vi "CurlingRobot_DrivingController_DGIST_ver.Manual.vi"() -> ()   [LabVIEW 2015]
uses:
  <vilib>/myRIO/Express VI/Onboard IO/AO/AO Express VI.xnode
  <vilib>/myRIO/Instrument Drivers/Onboard IO/AO/typedefs/AO Reference.ctl
  <vilib>/myRIO/Instrument Drivers/Onboard IO/AO/AO.lvlib
  <vilib>/myRIO/Common/Instrument Driver Framework/Utilities/typedefs/Analog Scaling Constants List.ctl
  <vilib>/myRIO/Common/Instrument Driver Framework/Utilities/typedefs/Analog Scaling Constants.ctl
  <vilib>/myRIO/Common/Instrument Driver Framework/myRIO v1.0/AO/typedefs/AO Channels List.ctl
  <vilib>/myRIO/Common/Instrument Driver Framework/myRIO v1.0/AO/typedefs/AO Channels Enum.ctl
  <vilib>/myRIO/Common/Instrument Driver Framework/Utilities/typedefs/myRIO Generic Hardware Reference.ctl
  <vilib>/myRIO/Common/Instrument Driver Framework/Utilities/typedefs/myRIO v1.0 Reference.ctl
  <vilib>/myRIO/Common/Instrument Driver Framework/Utilities/typedefs/Generic FPGA Reference.ctl
  <vilib>/myRIO/Common/Instrument Driver Framework/Utilities/typedefs/Hardware Version Enum.ctl
  <vilib>/myRIO/Instrument Drivers/Onboard IO/AO/vis/myRIO AO Open.xnode
  <vilib>/userdefined/High Color/nirio_resource_hc.ctl
  <vilib>/myRIO/Common/Instrument Driver Framework/myRIO v1.0/AO/vis/myRIO v1.1 Open AO.vi
  <vilib>/myRIO/Common/Instrument Driver Framework/Utilities/vis/Is FPGA Ref Available.vi
  <vilib>/platform/TimedLoop/XDataNode/XDataNode.xnode
  <vilib>/Platform/TimedLoop/XDataNode/timing_clust.ctl
  <vilib>/Platform/TimedLoop/XDataNode/XDNodeRunTimeDep.lvlib
  <vilib>/Platform/TimedLoop/XDataNode/wakeup.ctl
  <vilib>/Platform/TimedLoop/XDataNode/nitl_modes.ctl
  <vilib>/myRIO/Express VI/Onboard IO/Encoder/Encoder Express VI.xnode
  <vilib>/myRIO/Common/Instrument Driver Framework/myRIO v1.0/Encoder/typedefs/Encoder Count Direction Enum.ctl
  <vilib>/myRIO/Instrument Drivers/Onboard IO/Encoder/typedefs/Encoder Reference.ctl
  <vilib>/myRIO/Instrument Drivers/Onboard IO/Encoder/Encoder.lvlib
  <vilib>/myRIO/Common/Instrument Driver Framework/myRIO v1.0/Encoder/typedefs/Encoder Channels Enum.ctl
  <vilib>/myRIO/Common/Instrument Driver Framework/myRIO v1.0/Encoder/typedefs/Encoder Signal Mode.ctl
  <vilib>/myRIO/Instrument Drivers/Onboard IO/Encoder/vis/Read.vi
  <vilib>/myRIO/Instrument Drivers/Onboard IO/Encoder/vis/myRIO Encoder Open.xnode
  <vilib>/myRIO/Common/Instrument Driver Framework/myRIO v1.0/Encoder/typedefs/Encoder Configuration v1.0.ctl
  <vilib>/myRIO/Common/Instrument Driver Framework/myRIO v1.0/Encoder/vis/myRIO v1.1 Open Encoder.vi
  <vilib>/myRIO/Common/Instrument Driver Framework/myRIO v1.0/Encoder/vis/myRIO v1.0 Configure Encoder.vi
  <vilib>/myRIO/Express VI/Onboard IO/DO/DO Express VI.xnode
  <vilib>/myRIO/Instrument Drivers/Onboard IO/DIO/typedefs/DIO Reference.ctl
  <vilib>/myRIO/Instrument Drivers/Onboard IO/DIO/DIO.lvlib
  <vilib>/myRIO/Common/Instrument Driver Framework/myRIO v1.0/DIO/typedefs/DIO Channels List.ctl
  <vilib>/myRIO/Common/Instrument Driver Framework/myRIO v1.0/DIO/typedefs/DIO Channels Enum.ctl
  <vilib>/myRIO/Instrument Drivers/Onboard IO/DIO/vis/myRIO DIO Open.xnode
  <vilib>/myRIO/Common/Instrument Driver Framework/myRIO v1.0/DIO/vis/myRIO v1.1 Open DIO.vi
  <vilib>/myRIO/Instrument Drivers/Onboard IO/I2C/I2C.lvlib
  <vilib>/myRIO/Instrument Drivers/Onboard IO/I2C/typedefs/I2C User Configuration.ctl
  <vilib>/myRIO/Instrument Drivers/Onboard IO/I2C/typedefs/I2C Transfer Rate.ctl
  <vilib>/myRIO/Instrument Drivers/Utilities/Utilities.lvlib
  <vilib>/Instr/_visa.llb/VISA Configure Serial Port (Instr).vi
  <vilib>/myRIO/Express VI/Onboard Devices/LED/LED Express VI.xnode
panel:
  in  "ratelimit band 2":dbl=0.0007
  in  "ratelimit cut 2":dbl=20.0
  in  "yaw_ratelimit 2":dbl=0.03
  out "Kt 3":dbl=0.062 format="%#_13g"
  out "Kt 2":dbl=0.062 format="%#_13g"
  in  "Yaw Cont on/off":bool
  in  "Kt":dbl=0.062 format="%#_13g"
  in  "acc m/s^2 Target":dbl=1.0
  in  "YMO 2":bool
  in  "Reset":bool
  in  "Start":bool
  in  "enable":bool
  in  "vel_target":dbl=4.0
  in  "Angle":dbl
  out "now ang":dbl
  out "resetloop2":i32
  out "reset loop":i32=141402027
  in  "system off":bool
  out "mainloop":bool
  out "reset":bool
  out "outer loop time":i32
  in  "MFC":bool
  out "Wheel R_L velocity":cluster{dbl, dbl}(graph)={-1.1e-322, -1.6252354122998597e-232}
  in  "PD_cut_rot 2":dbl=500.0
  in  "Kp_rot 3":dbl=0.01
  in  "Kd_rot 4":dbl=0.0005
  out "ang_bias remover":dbl=180.0
  out "Abs angle or gyro":dbl=-0.00531
  in  "abs gy stop Button":bool
  in  "system off":bool
  in  "reset loop":bool
  out "vel_ref_velFB_YMOO":cluster{"V_in":dbl, dbl, "DOB FB":dbl}(graph)={"V_in"=8.658658111174331e-05, -1.5e-323, "DOB FB"=-0.0}
  in  "Mass":dbl=73.0
  out "now interation":i32
  in  "ratelimit band":dbl=0.0007
  in  "ratelimit cut":dbl=20.0
  in  "yaw_ratelimit":dbl=0.03
  out "time_now":u32=1627815
  out "tq in":dbl=0.000865321600614421
  out "Tq rot in":dbl
  out "DOB FB":dbl=-0.0
  out "Tq_inMFC":T1={"Numeric Control"=0.000865321600614421, "Numeric Control"=0.000865321600614421}
  out "Tq_in":T1={"Numeric Control"=0.000865321600614421, "Numeric Control"=0.000865321600614421}
  in  "Ki_longi":dbl=0.01
  in  "Kp_longi":dbl=10.0
  out "GyrowithHPF":dbl
  in  "Wheel Radius":dbl=0.125 format="%#_13g"
  out "V_wheel":dbl=-1.5e-323
  in  "Wheel B":dbl=1.0 format="%#_13g"
  in  "Wheel J":dbl=1.0 format="%#_13g"
  out "Wheel_OmegaL":dbl=-1.6252354122998597e-232
  out "Wheel_OmegaR":dbl=-1.1e-322
  out "Sampling Time":u32(graph)=1
  in  "MFC_FB_gain":dbl=2.0
  in  "MFC_HPF_cut":dbl=1.0
  in  "gy_offset_remover cutoff":dbl=0.05
  in  "PD on":bool
  in  "Kd_rot 3":dbl=0.003
  in  "Kp_rot 2":dbl=0.5
  in  "PD_cut_rot":dbl=30.0
  in  "FF_cut":dbl=3.0
  in  "DOB on":bool
  in  "DOB_FB_cut":dbl=16.0
  in  "Bm_rot":dbl=2.1
  in  "Jm_rot":dbl=0.6
  in  "Vel_cut":dbl=30.0
  out "Z rate":i16=79
  in  "[main loop]":bool
  # "longi vel cmd"
  # "MFC"
  # "Output"
  # "Longi vel control"
  # "Longi_ratelimeter"
  # "Yaw ref"
  # "Yaw control"
  # "Yaw  rate control"
  # "Dimension values"
  # "Gyro Filter setting"
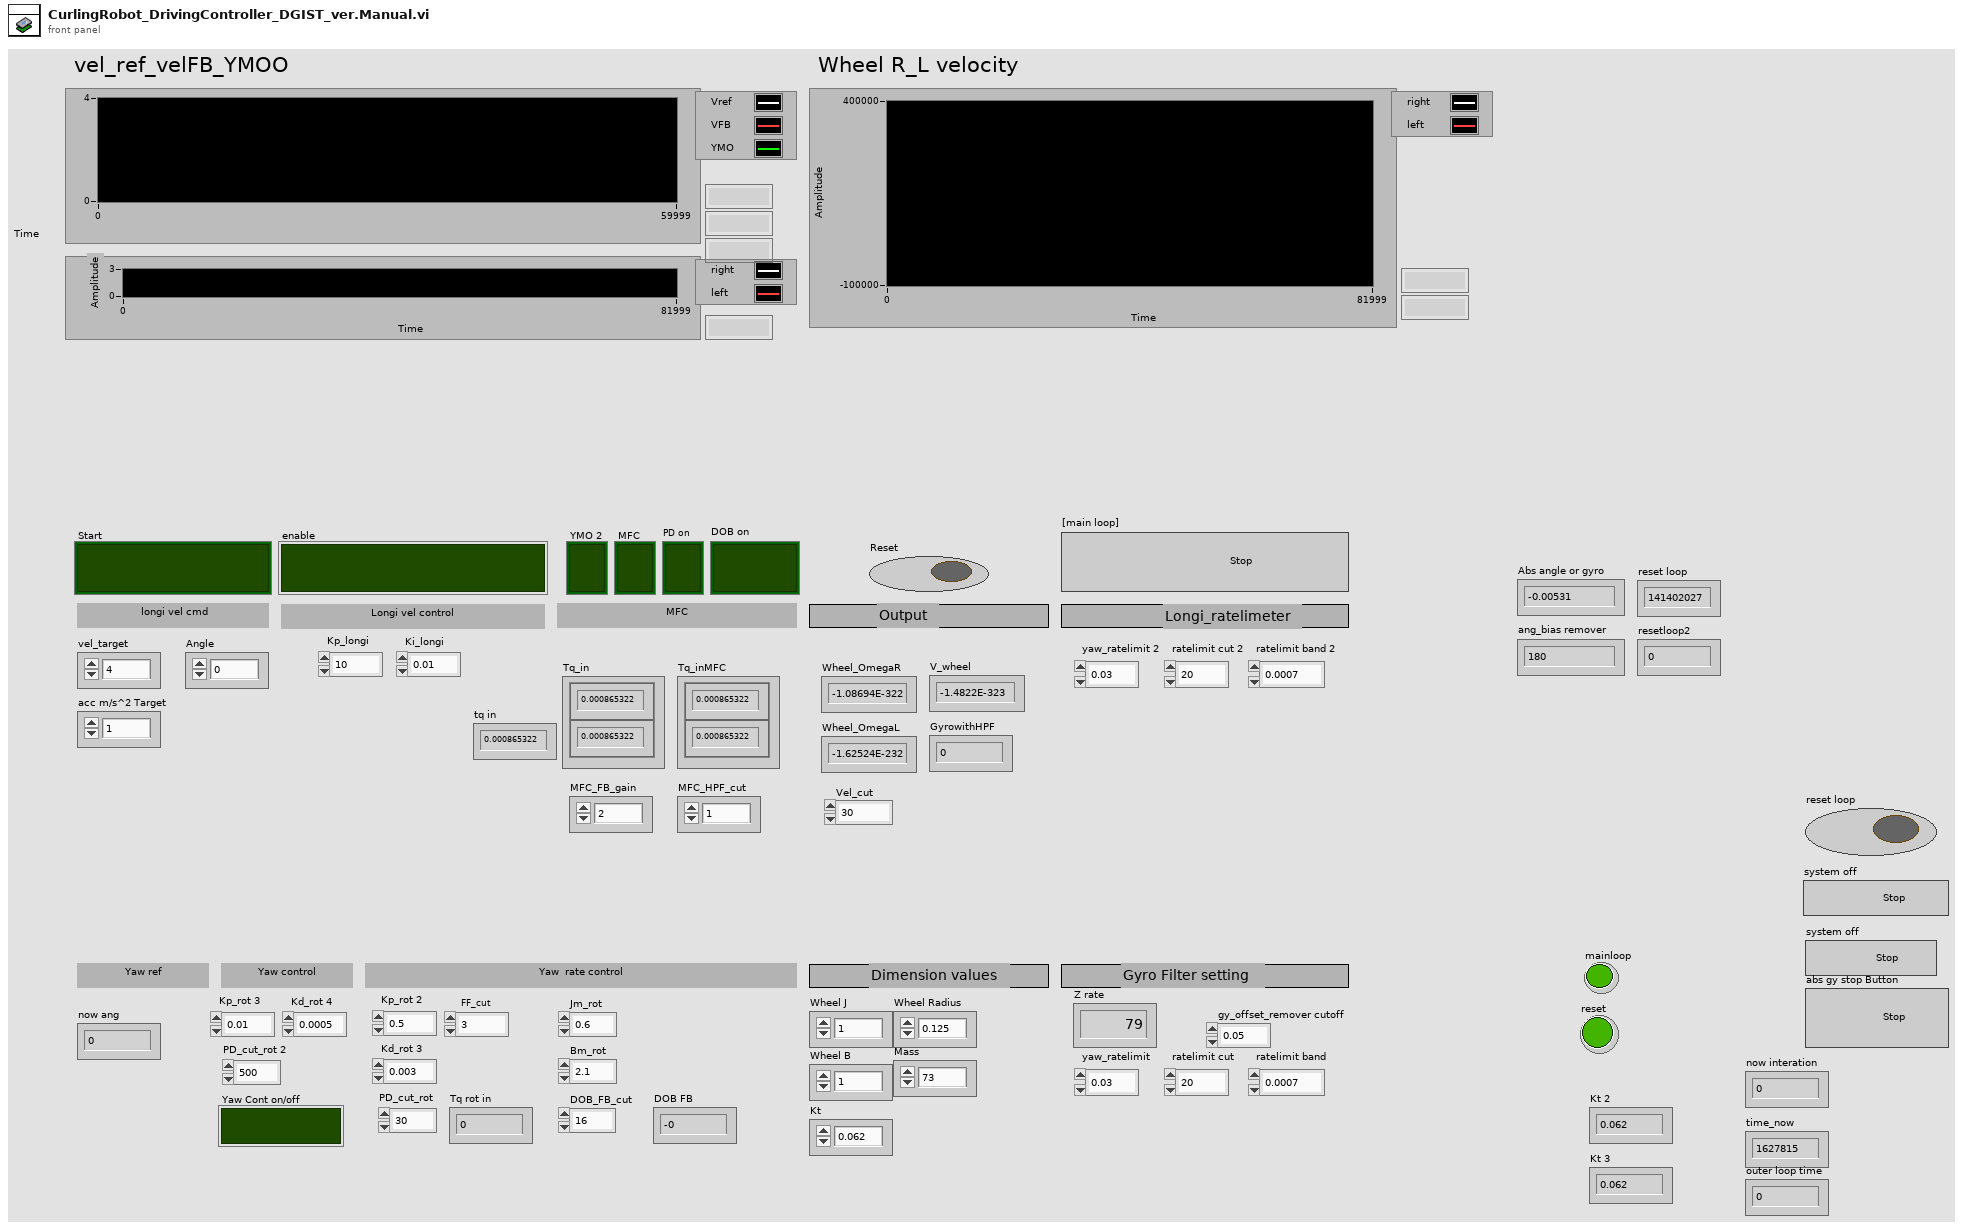
[diagram p1: front panel]
types:
  T1 = cluster{"Numeric Control":dbl, "Numeric Control":dbl}
  T2 = typedef "XDNodeRunTimeDep.lvlib/timing_clust.ctl" = cluster{"Expected End [f-1]":u64, "Actual End [f-1]":u64, "Finished Late? [f-1]":bool, "Expected End [i-1]":u64, "Actual End [i-1]":u64, "Finished Late? [i-1]":bool, "Expected Start [i]":u64, "Actual Start [i]":u64, "Expected Start [f]":u64, "Actual Start [f]":u64, "Source Name":string, "Structure Name":string, "Period":i64, "Deadline":i64, "Offset":i64, "Start":i64, "Priority":i32, "Timeout":i32, "Mode":T3, "Wakeup Reason":T4, "Error":errorcluster, "Source Type":string, "Secondary Source Type":string, "Global End Time":u64, "Global Start Time":u64, "Frame Duration":u64, "Iteration Duration":u64, "Assigned CPU":i32, "I/O Scan Engine Mode":u32}
  T3 = typedef "XDNodeRunTimeDep.lvlib/nitl_modes.ctl" = enum32{"No Change", "Process missed periods, maintain original phase", "Discard missed periods, maintain original phase", "Process missed periods, ignore original phase", "Discard missed periods, ignore original phase"}
  T4 = typedef "XDNodeRunTimeDep.lvlib/wakeup.ctl" = enum32{"Normal", "Aborted", "Asynchronous wakeup", "Timing source error", "Timed loop error", "Timeout"}
  T5 = typedef "DIO.lvlib/DIO Reference.ctl" = cluster{"myRIO Reference":T6, "DIO Channels List":T10}
  T6 = typedef "myRIO Generic Hardware Reference.ctl" = cluster{"myRIO Model":T7, "myRIO Hardware Reference":T8}
  T7 = typedef "Hardware Version Enum.ctl" = enum16{"Unknown", "myRIO-1900", "myRIO-1950", "roboRIO"}
  T8 = typedef "myRIO v1.0 Reference.ctl" = cluster{"Generic FPGA Reference":T9, "Allow multiple opens":bool}
  T9 = typedef "Generic FPGA Reference.ctl" = refnum<k20>
  T10 = typedef "DIO Channels List.ctl" = T11[]
  T11 = typedef "DIO Channels Enum.ctl" = enum16{"Not Connected", "C/DIO0", "C/DIO1", "C/DIO2", "C/DIO3", "C/DIO4", "C/DIO5", "C/DIO6", "C/DIO7", "A/DIO0", "A/DIO1", "A/DIO2", "A/DIO3", "A/DIO4", "A/DIO5", "A/DIO6", "A/DIO7", "A/DIO8", "A/DIO9", "A/DIO10", "A/DIO11", "A/DIO12", "A/DIO13", "A/DIO14", "A/DIO15", "B/DIO0", "B/DIO1", "B/DIO2", "B/DIO3", "B/DIO4", "B/DIO5", "B/DIO6", "B/DIO7", "B/DIO8", "B/DIO9", "B/DIO10", "B/DIO11", "B/DIO12", "B/DIO13", "B/DIO14", "B/DIO15", "LED0", "LED1", "LED2", "LED3", "Button0", "DIO/DIO0", "DIO/DIO1", "DIO/DIO2", "DIO/DIO3", "DIO/DIO4", "DIO/DIO5", "DIO/DIO6", "DIO/DIO7", "DIO/DIO8", "DIO/DIO9", "SPI/CS0", "SPI/CS1", "SPI/CS2", "SPI/CS3", "LED RADIO (Green)", "LED RADIO (Red)", "LED COMM (Green)", "LED COMM (Red)", "LED MODE (Green)", "LED MODE (Red)"}
  T12 = typedef "nirio_resource_hc.ctl" = tag
  T13 = typedef "Encoder.lvlib/Encoder Reference.ctl" = cluster{"myRIO Reference":T6, "Encoder Channels Enum":T14}
  T14 = typedef "Encoder Channels Enum.ctl" = enum16{"Not Connected", "C/ENC0", "C/ENC1", "A/ENC", "B/ENC", "DIO/ENC0", "DIO/ENC1", "DIO/ENC2", "DIO/ENC3", "DIO/ENC4"}
  T15 = typedef "Encoder Signal Mode.ctl" = enum16{"Quadrature phase signal", "Step and direction signal"}
  T16 = typedef "AO.lvlib/AO Reference.ctl" = cluster{"myRIO Reference":T6, "AO Channel List":T17, "AO Scaling Constant List":T19}
  T17 = typedef "AO Channels List.ctl" = T18[]
  T18 = typedef "AO Channels Enum.ctl" = enum16{"Not Connected", "AudioOut/Left", "AudioOut/Right", "C/AO0", "C/AO1", "A/AO0", "A/AO1", "B/AO0", "B/AO1"}
  T19 = typedef "Analog Scaling Constants List.ctl" = T20[]
  T20 = typedef "Analog Scaling Constants.ctl" = cluster{"LSB Weight (Volts)":dbl, "Offset (Volts)":dbl, "Signed?":bool}
  T21 = cluster{"baud rate (9600)":u32, "data bits (8)":u16, "parity (0:none)":enum16{"None", "Odd", "Even", "Mark", "Space"}, "stop bits (10: 1 bit)":u16, "flow control (0:none)":u16, "termination char\n(0xA = '\\n' = LF) ":u8, "Enable Termination\nChar (T)":bool, "timeout (10sec)":u32}
  T22 = typedef "I2C.lvlib/I2C User Configuration.ctl" = cluster{"I2C Transfer Rate":T23}
  T23 = typedef "I2C.lvlib/I2C Transfer Rate.ctl" = enum16{"Standard mode (100 kbps)", "Fast mode (400 kbps)"}
  T24 = typedef "I2C.lvlib/I2C Reference.ctl" = cluster{"myRIO Reference":T6, "I2C Channels Enum":T25, "I2C Configuration":T26}
  T25 = typedef "I2C Channels Enum.ctl" = enum16{"Not Connected", "A/I2C", "B/I2C", "I2C/I2C"}
  T26 = typedef "I2C.lvlib/I2C Configuration.ctl" = cluster{"I2C Transfer Rate":T23}
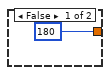
[diagram p7: hidden frame]
diagram:
  n1 = flat-sequence {
    frame #0 {
      n2 = node-c288() -> (w2:T2)  [unwired: 4 in]
      n3 = timed-loop {
        timing: w2 -> [_]
        timing-out: [_] -> w1
        i -> [w4]
        stop <- w6 stop-if-true
        w3 = 0 ("outer loop time 2")
        n4 = node-c288() -> ()  [unwired: 1 in, 1 out]
        n5 = local write "outer loop time"(w3) -> ()
        n6 = Greater?(x=w4, y=3.0) -> (0:w6:bool)
        n7 = local write "time_now"(w3) -> ()
        n8 = node-c288() -> ()  [unwired: 1 in, 1 out]
      }
      n9 = node-c288(w1) -> ()  [unwired: 1 out]
    }
    frame #1 {
      w12 = T21 {"baud rate (9600)"=38400, "data bits (8)"=8, "parity (0:none)"=enum."None", "stop bits (10: 1 bit)"=10, "flow control (0:none)"=0, "termination char\n(0xA = '\\n' = LF) "=10, "Enable Termination\nChar (T)"=TRUE, "timeout (10sec)"=10000}  # VISA Configuration
      w11 = refnum<visa-resource-name> "ASRL1::INSTR"  # VISA resource name in
      w32 = T22 {"I2C Transfer Rate"=enum."Fast mode (400 kbps)"}  # I2C bus speed
      w31 = tag "A/I2C"  # I2C channel
      w38 = u8 105  # PmodGYRO address
      # "Enable INT1 & \"data ready\" interrupt on INT2 pin"
      # "CTRL_REG3"
      # "Select HPF cutoff frequency"
      # "CTRL_REG2"
      # "Output select for LPF/HPF (both bypassed)"
      # "CTRL_REG5"
      # "Initialize device"
      # "Select data rate and enable measurements"
      # "Z-axis HI threshold"
      # "Enable interrupt on Z greater than HI threshold"
      # "CTRL_REG1"
      # "INT1_THS_ZH"
      # "INT1_CFG"
      # "Full scale setting = 100 dps"
      # "CTRL_REG4"
      # "register / data"
      n10 = while {
        i -> [w41]
        stop <- "system off" stop-if-true
        n11 = feedback #1(0) -> (w43:i32)
        n12 = case shown="False" "Reset" {
          tunnel: [w60 w61] -> w45
          tunnel: w41 -> [w60 _]
          tunnel: w43 -> [_ w61]
          frame False {
          }
          frame True {
          }
        }
        n13 = feedback-in #1(w45) -> ()
        n14 = Subtract(x=w41, y=w45) -> (x-y=w46:i32)
        "resetloop2" <- w46
        n15 = case shown="True" "Reset" {
          tunnel: w46 -> [_ w59]
          frame False {
          }
          frame True {
            n16 = Divide(x=w59, y=10000) -> (x/y=w51:dbl)
            n17 = Greater?(x=w51, y=1.0) -> (0:w54:bool)
            n18 = Greater?(x=w51, y=2.0) -> (0:w49:bool)
            n19 = Less?(x=w51, y=3.0) -> (x < y?=w53:bool)
            n20 = Less?(x=w51, y=4.0) -> (x < y?=w48:bool)
            n21 = And(x=w49, y=w48) -> (x .and. y?=w47:bool)
            "mainloop" <- w47
            n22 = local write "[main loop]"(w47) -> ()
            n23 = And(x=w54, y=w53) -> (x .and. y?=w52:bool)
            "reset" <- w52
            n24 = local write "reset loop"(w52) -> ()
            "outer loop time" <- w59
          }
        }
        "reset loop" <- w41
      }
      n25 = Unbundle By Name(w12) -> ("Enable Termination\nChar (T)"=w15:bool, "termination char\n(0xA = '\\n' = LF)"=w16:u8, "timeout (10sec)"=w17:u32, "baud rate (9600)"=w22:u32, "data bits (8)"=w21:u16, "parity (0:none)"=w20:enum16{"None", "Odd", "Even", "Mark", "Space"}, "stop bits (10: 1 bit)"=w19:u16, "flow control (0:none)"=w18:u16)
      n26 = call <vilib>:"Open.vi"("Channel Name"=w31) -> ("error out"=w34:errorcluster, "I2C Ref Out"=w33:T24)  [unwired: 9 in]
      n27 = node-c288() -> (w24:T2)  [unwired: 4 in]
      n28 = call-poly "VISA Configure Serial Port"("VISA resource name"=w11, "timeout (10sec)"=w17, "termination char\n(0xA = '\\n' = LF)"=w16, "Enable Termination\nChar (T)"=w15, "baud rate (9600)"=w22, "data bits (8)"=w21, "parity (0:none)"=w20, "stop bits (10: 1 bit)"=w19, "flow control (0:none)"=w18) -> ("VISA resource name out"=w13:refnum<visa-resource-name>, "error out"=w14:errorcluster)  [unwired: 5 in]
      n29 = call <vilib>:"Configure.vi"("error in (no error)"=w34, "I2C User Configuration"=w32, "I2C Ref In"=w33) -> ("error out"=w37:errorcluster, "I2C Ref Out"=w36:T24)  [unwired: 7 in]
      n30 = timed-loop {
        tunnel: w13 -> [w72]
        tunnel: w14 -> [w71]
        timing: w24 -> [_]
        timing-out: [_] -> w23
        stop <- "abs gy stop Button" stop-if-true
        w69 = u32 128  # 바이트 카운트
        n31 = node-c288() -> ()  [unwired: 1 in, 1 out]
        n32 = property class="Instr" props=["Serial Settings:Number of Bytes at Serial Port"](reference=w72) -> (reference out=w70:refnum<visa-resource-name>)  [unwired: 1 in, 2 out]
        n33 = call <vilib>:"Space Constant.vi"() -> ("String"=w65:string)
        n34 = VISA Read(VISA resource name=w70, byte count=w69, error in (no error)=w71) -> (read buffer=w68:string)  [unwired: 3 out]
        n35 = call <vilib>:"Trim Whitespace.vi"("string"=w68) -> ("trimmed string"=w67:string)  [unwired: 1 in]
        n36 = Match Pattern(string=w67, regular expression=w65) -> (before substring=w66:string)  [unwired: 1 in, 3 out]
        n37 = call <vilib>:"Trim Whitespace.vi"("string"=w66) -> ("trimmed string"=w64:string)  [unwired: 1 in]
        n38 = Fract/Exp String To Number(string=w64) -> (number=→"Abs angle or gyro":dbl)  [unwired: 3 in, 1 out]
        n39 = node-c288() -> ()  [unwired: 1 in, 1 out]
      }
      n40 = for {
        tunnel: [w696] -> w28
        tunnel: [w695] -> w27
        tunnel: [w691] -> w29
        tunnel: u8[][] [[34, 136], [35, 0], [48, 32], [54, 80], [36, 0], [33, 9], [32, 15]] ("Bytes to Write") -> [w694] mode=indexing
        tunnel: w36 -> [w693]
        tunnel: w37 -> [w692]
        tunnel: w38 -> [w691]
        n41 = call <vilib>:"Write.vi"("error in (no error)"=w692, "Bytes to Write"=w694, "Slave Address (7-bit)"=w691, "I2C Ref In"=w693) -> ("error out"=w696:errorcluster, "I2C Ref Out"=w695:T24)  [unwired: 6 in]
      }
      n42 = node-c288() -> (w26:T2)  [unwired: 4 in]
      n43 = node-c288(w23) -> ()  [unwired: 1 out]
      n44 = timed-loop {
        tunnel: w27 -> [w81]
        tunnel: w28 -> [w80]
        tunnel: w29 -> [w78]
        tunnel: [w79] -> w30
        timing: w26 -> [_]
        timing-out: [_] -> w25
        stop <- "system off" stop-if-true
        # "Integrate rate to obtain position"
        n45 = node-c288() -> ()  [unwired: 1 in, 1 out]
        n46 = case shown="False" "reset loop" {
          tunnel: w81 -> [w88 _]
          tunnel: w80 -> [w87 w688]
          tunnel: [w86 w688] -> w79
          tunnel: w78 -> [w85 _]
          frame False {
            n47 = node-c288() -> (w90:T2)  [unwired: 4 in]
            n48 = timed-loop {
              timing: w90 -> [_]
              timing-out: [_] -> w89
              tunnel: w88 -> [w202]
              tunnel: w87 -> [w201]
              tunnel: [w199] -> w86
              tunnel: w85 -> [w200]
              i -> [w284]
              stop <- "[main loop]" stop-if-true
              w157 = 0.0
              w192 = 0.0
              w218 = 0.0993 ("y")
              w279 = 0.0
              w408 = 0.001 ("input variable")
              w339 = 0.0 ("y0")
              w432 = 0.001 ("input variable")
              # "Longi velocity rate limiter"
              # "rated limiter"
              # "When stoppping LPF"
              # "angle limit +-90"
              # "To make zero angle"
              # "YR_ref"
              # "Read three 16-bit gyroscope values:\nWrite the address of the first register with MSB set to enable auto-indexing and then read six bytes"
              # "Format the six bytes into three 16-bit integers"
              # "calculatefixed offset"
              # "Rate limiter"
              # "rated limiter"
              # "save Drive time"
              # "when button start and stop within dive time automatly"
              # "Data saving"
              # "Longi velocity Plan"
              # "Longitudinal PI  controller"
              # "V longi FB"
              # "Tq longi in"
              # "Vel output"
              # "Tq rot in"
              # "Tq rot in"
              # "Gyro FB"
              # "Tq rot in"
              # "DOB FB"
              # "FF"
              # "Gyro FB"
              # "YMObser"
              # "Jacobian Robot to Wheel\nAnd (YMO FF FB) On off"
              # "YMO controller"
              # "Jacobian Wheel to robot"
              # "Wheel MFC controller"
              # "MFC_HPF"
              # "MFC controller ModelEuler not Tustin"
              # "Tq_Right"
              # "Tq_Left"
              # "Time derivative of enc to gel wheel vel"
              # "Wheel encoder gear ratio, encoder"
              # "MFC_HPF"
              # "MFC controller ModelEuler not Tustin"
              # "Rot PD  controller"
              # "gear ratio"
              # "gear ratio"
              n49 = node-c288() -> ()  [unwired: 1 in, 1 out]
              n50 = local read "ang_bias remover"() -> (w176:dbl)
              n51 = local read "now interation"() -> (w163:i32)
              n52 = local read "now interation"() -> (w234:i32)
              n53 = Greater?(x=w163, y=15000) -> (0:w153:bool)
              n54 = Greater?(x=w163, y=14000) -> (0:w149:bool)
              n55 = Greater?(x=w163, y=16000) -> (0:w154:bool)
              n56 = formula code="float phi_cmd;\nif (ref_phi >= 70)\nphi_cmd = 70;\nelse if (ref_phi <= -70)\nphi_cmd = -70;\nelse\nphi_cmd = ref_phi;"("ref_phi"="Angle") -> ("phi_cmd"=w179:dbl)
              n57 = Divide(x=w234, y=u32 1000) -> (x/y=w135:dbl)
              n58 = feedback #2(w157) -> (w160:dbl)
              n59 = case shown="False" w149 {
                tunnel: w176 -> [w487 _]
                tunnel: [w487 w488] -> w150
                tunnel: w160 -> [_ w488]
                frame False {
                }
                frame True {
                }
              }
              n60 = feedback-in #2(w150) -> ()
              n61 = feedback #3(w157) -> (w158:dbl)
              n62 = case shown="False" w154 {
                tunnel: w176 -> [w483 _]
                tunnel: [w483 w484] -> w156
                tunnel: w158 -> [_ w484]
                frame False {
                }
                frame True {
                }
              }
              n63 = feedback-in #3(w156) -> ()
              n64 = feedback #4(w157) -> (w159:dbl)
              n65 = case shown="False" w153 {
                tunnel: w176 -> [w485 _]
                tunnel: [w485 w486] -> w155
                tunnel: w159 -> [_ w486]
                frame False {
                }
                frame True {
                }
              }
              n66 = feedback-in #4(w155) -> ()
              n67 = Compound Arithmetic op=ADD(w158, w159, w160) -> (w161:dbl)
              n68 = Divide(x=w161, y=3.0) -> (x/y=w164:dbl)
              n69 = Subtract(x=w176, y=w164) -> (x-y=w178:dbl)
              "now ang" <- w178
              n70 = formula code="float phi;\nif (sensor > 90 && sensor <=270)\nphi = 180-sensor;\nelse if (sensor >270)\nphi = sensor - 360;\nelse\nphi = sensor;"("sensor"=w178) -> ("phi"=w177:dbl)
              n71 = Negate(x=w177) -> (-x=w182:dbl)
              n72 = Bundle(w179, w182) -> ()  [unwired: 1 in, 1 out]
              n73 = Subtract(x=w179, y=w182) -> (x-y=w180:dbl)
              n74 = Add(x=w180, y=0.0) -> (x+y=w181:dbl)
              n75 = feedback #5(0.0) -> (w169:dbl)
              n76 = feedback-in #5(w181) -> ()
              n77 = call <vilib>:"Write Read.vi"("Byte Count"=u32 6, "error in (no error)"=w201, "Bytes to Write"=u8[] [168], "Slave Address (7-bit)"=w200, "I2C Ref In"=w202) -> ("error out"=w199:errorcluster, "Bytes Read"=w217:u8[])  [unwired: 3 in, 1 out]
              n78 = Index Array "Index Array"(array=w217) -> (element #1=w212:u8, element #2=w211:u8, element #3=w210:u8, element #4=w209:u8, element #5=w208:u8, element #6=w207:u8)  [unwired: 6 in]
              n79 = Multiply(x="PD_cut_rot 2", y=6.283185307179586) -> (x*y=w166:dbl)
              n80 = Join Numbers(hi=w211, lo=w212) -> ((hi.lo)=w215:u16)
              n81 = Join Numbers(hi=w209, lo=w210) -> ((hi.lo)=w214:u16)
              n82 = Join Numbers(hi=w207, lo=w208) -> ((hi.lo)=w213:u16)
              n83 = Reciprocal(x=w166) -> (1/x=w167:dbl)
              n84 = feedback #6(0.0) -> (w173:dbl)
              n85 = formula code="float F,A,B,C,ykd,ykp,y0;\nF=2*tau+T;\nA=(2*Kd_rot)/F;\nB=(-2*Kd_rot)/F;\nC=(2*tau-T)/F;\nykd=A*u0+B*u1+C*y1;\nykp=Kp_rot*u0;\ny0=ykp+ykd;"("tau"=w167, "u0"=w181, "u1"=w169, "y1"=w173, "T"=0.001 ("input variable"), "Kp_rot"="Kp_rot 3", "Kd_rot"="Kd_rot 4") -> ("y0"=w183:dbl)
              n86 = feedback-in #6(w183) -> ()
              n87 = To Word Integer(number=w215) -> ()  [unwired: 1 out]
              n88 = To Word Integer(number=w214) -> ()  [unwired: 1 out]
              n89 = To Word Integer(number=w213) -> (16bit integer=w216:i16)
              "Z rate" <- w216
              n90 = Add(x=0.0, y=w183) -> (x+y=w123:dbl)
              n91 = feedback #7(0.0) -> (w272:dbl)
              n92 = case shown="True" "Start" {
                tunnel: w135 -> [w540 _]
                tunnel: [w540 w541] -> w271
                tunnel: w272 -> [_ w541]
                frame False {
                }
                frame True {
                }
              }
              n93 = feedback-in #7(w271) -> ()
              n94 = Divide(x=w216, y=65535.0 ("gyroscale")) -> (x/y=w203:dbl)
              n95 = Subtract(x=w135, y=w271) -> (x-y=w131:dbl)
              n96 = formula code="float V_now;\nV_now=acc_d*t;\n\nif (V_now < V_targ && V_targ >= 0)\nV_in=V_now;\nelse if (V_targ < 0 && -V_now > V_targ )\nV_in=-V_now;\nelse \nV_in=V_targ;"("V_targ"="vel_target", "acc_d"="acc m/s^2 Target", "t"=w131) -> ("V_in"=w239:dbl)
              n97 = Select(t=w123, s="Yaw Cont on/off", f=0.0) -> (s? t:f=w122:dbl)
              n98 = feedback #8(0.0 ("V_in")) -> (w246:dbl)
              n99 = feedback-in #8(w239) -> ()
              n100 = Multiply(x=0.1, y=6.283185307179586) -> (x*y=w243:dbl)
              n101 = Reciprocal(x=w243) -> (1/x=w247:dbl)
              n102 = Multiply(x="PD_cut_rot", y=6.283185307179586) -> (x*y=w383:dbl)
              n103 = feedback #9(0.0) -> (w244:dbl)
              n104 = formula code="float F,A,B,C,y0;\nF=2*tau+T;\nA=(2*a+b*T)/F;\nB=(b*T-2*a)/F;\nC=(2*tau-T)/F;\ny0=A*u0+B*u1+C*y1;"("tau"=w247, "u0"=w239, "u1"=w246, "y1"=w244, "T"=0.001 ("input variable"), "a"=0.0 ("input variable"), "b"=1.0 ("input variable")) -> ("y0"=w236:dbl)
              n105 = case shown="False" "Start" {
                tunnel: [w538 w539] -> w118
                tunnel: w239 -> [_ w539]
                tunnel: w236 -> [w538 _]
                frame False {
                }
                frame True {
                }
              }
              n106 = feedback-in #9(w236) -> ()
              n107 = feedback #10(0.0) -> (w380:dbl)
              n108 = local read "DOB FB"() -> (w119:dbl)
              n109 = Reciprocal(x=w383) -> (1/x=w382:dbl)
              n110 = Multiply(x="FF_cut", y=6.283185307179586) -> (x*y=w405:dbl)
              n111 = feedback #11(0.0 ("gy_z[]")) -> (w393:dbl)
              n112 = feedback-in #11(w122) -> ()
              n113 = Reciprocal(x=w405) -> (1/x=w403:dbl)
              n114 = local read "Jm_rot"() -> (w314:dbl)
              n115 = feedback #12(0.0) -> (w108:dbl)
              n116 = Divide(x=w314, y=w218) -> (x/y=w313:dbl)
              n117 = local read "Bm_rot"() -> (w312:dbl)
              n118 = feedback #13(0.0) -> (w306:dbl)
              n119 = Divide(x=w312, y=w218) -> (x/y=w311:dbl)
              n120 = Multiply(x="ratelimit cut 2", y=6.283185307179586) -> (x*y=w106:dbl)
              n121 = Reciprocal(x=w106) -> (1/x=w105:dbl)
              n122 = feedback #14(0.0 ("gy_z[]")) -> (w402:dbl)
              n123 = formula code="float F,A,B,C,y0;\nF=2*tau+T;\nA=(2*a+b*T)/F;\nB=(b*T-2*a)/F;\nC=(2*tau-T)/F;\ny0=A*u0+B*u1+C*y1;"("tau"=w403, "u0"=w122, "u1"=w393, "y1"=w402, "T"=0.001 ("input variable"), "a"=w313, "b"=w311) -> ("y0"=w374:dbl)
              n124 = feedback-in #14(w374) -> ()
              n125 = feedback #15() -> (w375:dbl)  [unwired: 1 in]
              n126 = feedback #16(0.0) -> (w103:dbl)
              n127 = feedback #17(0.0 ("gy_ratelimit")) -> (w110:dbl)
              n128 = xnode "Digital output (1 sample)"("C/DIO1 (DIO1)"="enable") -> ()  [unwired: 1 in, 1 out]
              n129 = xnode "Left encoder"() -> ("Counter Value"=w139:i32)  [unwired: 2 in, 3 out]
              n130 = xnode "Encoder"() -> ("Counter Value"=w145:i32)  [unwired: 2 in, 3 out]
              n131 = Negate(x=w139) -> (-x=w138:i32)
              n132 = Negate(x=w145) -> (-x=w144:i32)
              n133 = Multiply(x=w138, y=6.283185307179586) -> (x*y=w443:dbl)
              n134 = Negate(x=w144) -> (-x=w441:i32)
              n135 = Divide(x=w443, y=32768.0) -> (x/y=w425:dbl)
              n136 = Multiply(x=w441, y=6.283185307179586) -> (x*y=w446:dbl)
              n137 = feedback #18(0.0 ("f")) -> (w224:dbl)
              n138 = Multiply(x=2.0 ("y"), y=w224) -> (x*y=w226:dbl)
              n139 = Divide(x=w446, y=32768.0) -> (x/y=w342:dbl)
              n140 = feedback #19(0.0) -> (w410:dbl)
              n141 = feedback #20(0.0 ("gy_z[]")) -> (w407:dbl)
              n142 = local read "Wheel Radius"() -> (w297:dbl)
              n143 = Bundle(w342, w425) -> (w422:cluster{dbl, dbl})  [unwired: 1 in]
              n144 = feedback #21(0.0 ("f")) -> (w222:dbl)
              n145 = Multiply(x=2.0 ("y"), y=w222) -> (x*y=w221:dbl)
              n146 = local read "Kt"() -> (w125:dbl)
              "Kt 3" <- w125
              n147 = feedback #22(0.0 ("gy_ratelimit")) -> (w266:dbl)
              n148 = local read "now interation"() -> (w134:i32)
              n149 = Divide(x=w422, y=8.0) -> (x/y=w296:cluster{dbl, dbl})
              n150 = Multiply(x=w296, y=w297) -> (x*y=w116:cluster{dbl, dbl})
              n151 = Divide(x="Jm_rot", y=w125) -> (x/y=w401:dbl)
              n152 = Multiply(x="DOB_FB_cut", y=6.283185307179586) -> (x*y=w411:dbl)
              n153 = Unbundle(w116) -> ()  [unwired: 2 out]
              n154 = Reciprocal(x=w411) -> (1/x=w413:dbl)
              n155 = feedback #23(0.0) -> (w259:dbl)
              n156 = feedback #24(0.0) -> (w436:dbl)
              n157 = feedback-in #24(w342) -> ()
              n158 = Divide(x="Bm_rot", y=w125) -> (x/y=w400:dbl)
              n159 = feedback #25(0.0) -> (w429:dbl)
              n160 = feedback-in #25(w425) -> ()
              n161 = feedback #26(0.0) -> (w328:dbl)
              n162 = feedback #27(0.0) -> (w353:dbl)
              n163 = local read "Abs angle or gyro"() -> (w187:dbl)
              n164 = Multiply(x="MFC_HPF_cut", y=6.283185307179586) -> (x*y=w355:dbl)
              n165 = Multiply(x="ratelimit cut", y=6.283185307179586) -> (x*y=w262:dbl)
              n166 = Reciprocal(x=w355) -> (1/x=w322:dbl)
              n167 = Greater?(x=w134, y=2000) -> (0:w197:bool)
              n168 = Greater?(x=w134, y=12000) -> (0:w195:bool)
              n169 = Reciprocal(x=w262) -> (1/x=w261:dbl)
              n170 = Multiply(x="Vel_cut", y=6.283185307179586) -> (x*y=w434:dbl)
              n171 = feedback #28(0.0) -> (w409:dbl)
              n172 = feedback #29(0.0) -> (w406:dbl)
              n173 = Multiply(x="Vel_cut", y=6.283185307179586) -> (x*y=w439:dbl)
              n174 = Reciprocal(x=w434) -> (1/x=w431:dbl)
              n175 = Reciprocal(x=w439) -> (1/x=w438:dbl)
              n176 = feedback #30(0.0) -> (w264:dbl)
              n177 = feedback #31(0.0) -> (w361:dbl)
              n178 = feedback-in #31(w203) -> ()
              n179 = feedback #32(0.0) -> (w391:dbl)
              n180 = feedback #33(w192) -> (w194:dbl)
              n181 = case shown="True" w197 {
                tunnel: w187 -> [w501 _]
                tunnel: [w501 w502] -> w188
                tunnel: w194 -> [_ w502]
                frame False {
                }
                frame True {
                }
              }
              n182 = feedback-in #33(w188) -> ()
              n183 = Boolean To (0,1)(Boolean="DOB on") -> (0, 1=w397:i16)
              n184 = Multiply(x=w397, y=w391) -> (x*y=w307:dbl)
              "DOB FB" <- w307
              n185 = feedback #34(w339) -> (w430:dbl)
              n186 = formula code="y0=(2*(u0-u1)-(T-2*Tau)*y1)/(T+2*Tau);"("Tau"=w431, "u0"=w425, "u1"=w429, "y1"=w430, "T"=w432) -> ("y0"=w426:dbl)
              n187 = feedback-in #34(w426) -> ()
              n188 = feedback #35(w192) -> (w193:dbl)
              n189 = case shown="False" w195 {
                tunnel: w187 -> [w499 _]
                tunnel: [w499 w500] -> w189
                tunnel: w193 -> [_ w500]
                frame False {
                }
                frame True {
                }
              }
              n190 = feedback-in #35(w189) -> ()
              n191 = feedback #36(w339) -> (w437:dbl)
              n192 = formula code="y0=(2*(u0-u1)-(T-2*Tau)*y1)/(T+2*Tau);"("Tau"=w438, "u0"=w342, "u1"=w436, "y1"=w437, "T"=w432) -> ("y0"=w341:dbl)
              n193 = feedback-in #36(w341) -> ()
              n194 = feedback #37(0.0 ("y0")) -> (w330:dbl)
              n195 = feedback #38(0.0 ("y0")) -> (w351:dbl)
              n196 = Tick Count (ms)() -> (millisecond timer value=w344:u32)
              "time_now" <- w344
              n197 = Multiply(x="gy_offset_remover cutoff", y=6.283185307179586) -> (x*y=w366:dbl)
              n198 = feedback #39() -> (w343:u32)  [unwired: 1 in]
              n199 = feedback-in #39(w344) -> ()
              n200 = Subtract(x=w344, y=w343) -> (x-y=w115:u32)
              "Sampling Time" <- w115
              n201 = Reciprocal(x=w366) -> (1/x=w288:dbl)
              n202 = feedback #40(0.0) -> (w359:dbl)
              n203 = local read "Kt"() -> (w124:dbl)
              "Kt 2" <- w124
              n204 = feedback #41(0.0) -> (w334:dbl)
              n205 = Greater?(x=w134, y=13000) -> (0:w190:bool)
              n206 = Bundle("y0"=w341, "y0"=w426) -> (w340:cluster{"y0":dbl, "y0":dbl})  [unwired: 1 in]
              n207 = Divide(x=w340, y=8.0) -> (x/y=w112:cluster{"y0":dbl, "y0":dbl})
              "Wheel R_L velocity" <- w112
              n208 = case shown="True" w190 {
                tunnel: w189 -> [_ w498]
                tunnel: [180 w494] -> w186
                tunnel: w188 -> [_ w497]
                tunnel: w187 -> [_ w490]
                tunnel: w134 -> [_ w492]
                frame False {
                }
                frame True {
                  n209 = Subtract(x=w498, y=w497) -> (x-y=w496:dbl)
                  n210 = Divide(x=w496, y=10000) -> (x/y=w493:dbl)
                  n211 = Multiply(x=w493, y=w492) -> (x*y=w491:dbl)
                  n212 = Subtract(x=w490, y=w491) -> (x-y=w494:dbl)
                }
              }
              "ang_bias remover" <- w186
              n213 = feedback #42(0.0) -> (w365:dbl)
              n214 = formula code="float F,A,B,C,y0;\nF=2*tau+T;\nA=(2*a+b*T)/F;\nB=(b*T-2*a)/F;\nC=(2*tau-T)/F;\ny0=A*u0+B*u1+C*y1;"("tau"=w288, "u0"=w203, "u1"=w361, "y1"=w365, "T"=0.001 ("input variable"), "a"=0.0 ("input variable"), "b"=1.0 ("input variable")) -> ("y0"=w267:dbl)
              n215 = feedback-in #42(w267) -> ()
              n216 = Less?(x=w115, y=1.1) -> (x < y?=w113:bool)
              n217 = Unbundle(w112) -> ("y0"=→"Wheel_OmegaR":dbl, "y0"=→"Wheel_OmegaL":dbl)
              n218 = Unbundle(w296) -> ()  [unwired: 2 out]
              n219 = xnode "LED"("LED3"=w113) -> ()  [unwired: 1 in, 1 out]
              n220 = Greater?(x=w284, y=21000) -> (0:w283:bool)
              n221 = Greater?(x=w284, y=20000) -> (0:w289:bool)
              n222 = Greater?(x=w284, y=22000) -> (0:w282:bool)
              n223 = feedback #43(0.0 ("y0")) -> (w360:dbl)
              n224 = feedback #44(0.0 ("y0")) -> (w333:dbl)
              n225 = local read "Wheel_OmegaR"() -> (w111:dbl)
              n226 = local read "Wheel_OmegaL"() -> (w91:dbl)
              n227 = feedback #45(w279) -> (w276:dbl)
              n228 = case shown="False" w289 {
                tunnel: w267 -> [w546 _]
                tunnel: [w546 w547] -> w287
                tunnel: w276 -> [_ w547]
                frame False {
                }
                frame True {
                }
              }
              n229 = feedback-in #45(w287) -> ()
              n230 = feedback #46(w279) -> (w278:dbl)
              n231 = case shown="False" w282 {
                tunnel: w267 -> [w542 _]
                tunnel: [w542 w543] -> w280
                tunnel: w278 -> [_ w543]
                frame False {
                }
                frame True {
                }
              }
              n232 = feedback-in #46(w280) -> ()
              n233 = feedback #47(w279) -> (w277:dbl)
              n234 = case shown="False" w283 {
                tunnel: w267 -> [w544 _]
                tunnel: [w544 w545] -> w281
                tunnel: w277 -> [_ w545]
                frame False {
                }
                frame True {
                }
              }
              n235 = feedback-in #47(w281) -> ()
              n236 = Compound Arithmetic op=ADD(w278, w277, w276) -> (w275:dbl)
              n237 = Add(x=w111, y=w91) -> (x+y=w318:dbl)
              n238 = Divide(x=w275, y=3.0) -> (x/y=w250:dbl)
              n239 = Subtract(x=w203, y=w250) -> (x-y=w233:dbl)
              n240 = formula code="float rate;\nrate=gy-gy_r1;\nif (rate > limit)\ngy_ratelimit=gy_r1+limit;\nelse if (rate < -limit)\ngy_ratelimit=gy_r1+(-limit);\nelse\ngy_ratelimit=gy;"("gy"=w233, "gy_r1"=w266, "limit"="yaw_ratelimit") -> ("gy_ratelimit"=w249:dbl)
              n241 = feedback-in #22(w249) -> ()
              n242 = feedback-in #23(w249) -> ()
              n243 = formula code="float F,A,B,C,y0;\nF=2*tau+T;\nA=(2*a+b*T)/F;\nB=(b*T-2*a)/F;\nC=(2*tau-T)/F;\ny0=A*u0+B*u1+C*y1;"("tau"=w261, "u0"=w249, "u1"=w259, "y1"=w264, "T"=0.001 ("input variable"), "a"=0.0 ("input variable"), "b"=1.0 ("input variable")) -> ("y0"=w254:dbl)
              n244 = feedback-in #30(w254) -> ()
              n245 = formula code="float band_ratelim;\n\nif (gy_ratelim < gy_band && gy_ratelim > -gy_band)\nband_ratelim=0;\nelse\nband_ratelim=gy_ratelim;"("gy_ratelim"=w254, "gy_band"="ratelimit band") -> ("band_ratelim"=w137:dbl)
              "GyrowithHPF" <- w137
              n246 = Subtract(x=w122, y=w137) -> (x-y=w379:dbl)
              n247 = feedback-in #10(w379) -> ()
              n248 = formula code="float F,A,B,C,ykd,ykp,y0;\nF=2*tau+T;\nA=(2*Kd_rot)/F;\nB=(-2*Kd_rot)/F;\nC=(2*tau-T)/F;\nykd=A*u0+B*u1+C*y1;\nykp=Kp_rot*u0;\ny0=ykp+ykd;"("tau"=w382, "u0"=w379, "u1"=w380, "y1"=w375, "T"=0.001 ("input variable"), "Kp_rot"="Kp_rot 2", "Kd_rot"="Kd_rot 3") -> ("y0"=w371:dbl)
              n249 = feedback-in #15(w371) -> ()
              n250 = Select(t=w371, s="PD on", f=0.0) -> (s? t:f=w310:dbl)
              n251 = Add(x=w374, y=w310) -> (x+y=w147:dbl)
              n252 = Add(x=0.0, y=w147) -> (x+y=w146:dbl)
              n253 = Subtract(x=w146, y=w307) -> (x-y=w308:dbl)
              "Tq rot in" <- w308
              n254 = formula code="v_L=-error_YR/2;\n\nif (v_L < 16.5 && v_L > -16.5)\nv_L=v_L;\nelse if (v_L >=16.5)\nv_L=16.5;\nelse\nv_L=-16.5;\nv_R=error_YR/2;\n\nif (v_R < 16.5 && v_R > -16.5)\nv_R=v_R;\nelse if (v_R >=16.5)\nv_R=16.5;\nelse\nv_R=-16.5;"("error_YR"=w308) -> ("v_L"=w315:dbl, "v_R"=w316:dbl)
              n255 = feedback-in #19(w308) -> ()
              n256 = feedback-in #20(w137) -> ()
              n257 = formula code="float F,A,B,C,y0;\nF=2*tau+T;\nA=(2*a+b*T)/F;\nB=(b*T-2*a)/F;\nC=(2*tau-T)/F;\ny0=A*u0+B*u1+C*y1;"("tau"=w413, "u0"=w137, "u1"=w407, "y1"=w406, "T"=w408, "a"=w401, "b"=w400) -> ("y0"=w395:dbl)
              n258 = formula code="float F,A,B,C,y0;\nF=2*tau+T;\nA=(2*a+b*T)/F;\nB=(b*T-2*a)/F;\nC=(2*tau-T)/F;\ny0=A*u0+B*u1+C*y1;"("tau"=w413, "u0"=w308, "u1"=w410, "y1"=w409, "T"=w408, "a"=0.0 ("input variable"), "b"=1.0 ("input variable")) -> ("y0"=w399:dbl)
              n259 = feedback-in #28(w399) -> ()
              n260 = feedback-in #29(w395) -> ()
              n261 = Subtract(x=w395, y=w399) -> (x-y=w398:dbl)
              n262 = feedback-in #32(w398) -> ()
              n263 = Divide(x=w318, y=2.0) -> ()  [unwired: 1 out]
              n264 = Multiply(x=w91, y="Wheel Radius") -> (x*y=w93:dbl)
              "V_wheel" <- w93
              n265 = formula code="float rate;\nrate=gy-gy_r1;\nif (rate > limit)\ngy_ratelimit=gy_r1+limit;\nelse if (rate < -limit)\ngy_ratelimit=gy_r1+(-limit);\nelse\ngy_ratelimit=gy;"("gy"=w93, "gy_r1"=w110, "limit"="yaw_ratelimit 2") -> ("gy_ratelimit"=w94:dbl)
              n266 = formula code="float F,A,B,C,y0;\nF=2*tau+T;\nA=(2*a+b*T)/F;\nB=(b*T-2*a)/F;\nC=(2*tau-T)/F;\ny0=A*u0+B*u1+C*y1;"("tau"=w105, "u0"=w94, "u1"=w103, "y1"=w108, "T"=0.001 ("input variable"), "a"=0.0 ("input variable"), "b"=1.0 ("input variable")) -> ("y0"=w98:dbl)
              n267 = formula code="float band_ratelim;\n\nif (gy_ratelim < gy_band && gy_ratelim > -gy_band)\nband_ratelim=0;\nelse\nband_ratelim=gy_ratelim;"("gy_ratelim"=w98, "gy_band"="ratelimit band 2") -> ("band_ratelim"=w92:dbl)
              n268 = feedback-in #12(w98) -> ()
              n269 = Subtract(x=w118, y=w92) -> (x-y=w300:dbl)
              n270 = Bundle("V_in"=w118, w92) -> ()  [unwired: 1 in, 1 out]
              n271 = Bundle("V_in"=w118, w92, "DOB FB"=w119) -> (→"vel_ref_velFB_YMOO":cluster{"V_in":dbl, dbl, "DOB FB":dbl})  [unwired: 1 in]
              n272 = feedback-in #13(w300) -> ()
              n273 = formula code="float ykd,ykp,y0;\n\nykd=Kp*u0;\nykp=Ki*(u0-u1)/T;\ny0=ykp+ykd;"("u0"=w300, "u1"=w306, "T"=0.001 ("input variable"), "Kp"="Kp_longi", "Ki"="Ki_longi") -> ("y0"=w301:dbl)
              "tq in" <- w301
              n274 = feedback-in #16(w94) -> ()
              n275 = feedback-in #17(w94) -> ()
              n276 = case shown="True" "YMO 2" {
                tunnel: [w640 w645] -> w220
                tunnel: [w640 w644] -> w293
                tunnel: w316 -> [_ w643]
                tunnel: w315 -> [_ w642]
                tunnel: w301 -> [w640 w641]
                frame False {
                }
                frame True {
                  n277 = Add(x=w641, y=w643) -> (x+y=w645:dbl)
                  n278 = Add(x=w641, y=w642) -> (x+y=w644:dbl)
                }
              }
              n279 = Bundle(w220, w293) -> (→"Tq_in":cluster{dbl, dbl})  [unwired: 1 in]
              n280 = Subtract(x=w293, y=w221) -> (x-y=w292:dbl)
              n281 = Subtract(x=w220, y=w226) -> (x-y=w219:dbl)
              n282 = Bundle(w219, w292) -> (→"Tq_inMFC":cluster{dbl, dbl})  [unwired: 1 in]
              n283 = Negate(x=w219) -> (-x=w421:dbl)
              n284 = Bundle(w220, w219) -> ()  [unwired: 1 in, 1 out]
              n285 = Divide(x=w292, y=1.0) -> (x/y=w141:dbl)
              n286 = Divide(x=w421, y=1.0) -> (x/y=w143:dbl)
              n287 = Negate(x=w141) -> (-x=w140:dbl)
              n288 = Negate(x=w143) -> (-x=w142:dbl)
              n289 = xnode "Analog output (1 sample) 4"("C/AO1 (AO1)"=w142, "C/AO0 (AO0)"=w140) -> ()  [unwired: 1 in, 1 out]
              n290 = feedback-in #40(w219) -> ()
              n291 = feedback-in #41(w292) -> ()
              n292 = formula code="float F,y0,B,J;\nJ=(Jw/2+Ma/2*r*r)/Kt;\nB=Bw/Kt;\nF=2*J+B*T;\ny0=(T*u0+T*u1+(2*J-B*T)*y1)/F;"("Jw"="Wheel J", "u0"=w219, "u1"=w359, "y1"=w360, "T"=0.001 ("input variable"), "Bw"="Wheel B", "Kt"="Kt", "Ma"="Mass", "r"="Wheel Radius") -> ("y0"=w228:dbl)
              n293 = formula code="float J,B,F,y0;\nJ=(Jw/2+Ma/2*r*r)/Kt;\nB=Bw/Kt;\nF=2*J+B*T;\ny0=(T*u0+T*u1+(2*J-B*T)*y1)/F;"("Jw"="Wheel J", "u0"=w292, "u1"=w334, "y1"=w333, "T"=0.001 ("input variable"), "Bw"="Wheel B", "Kt"=w124, "Ma"="Mass", "r"="Wheel Radius") -> ("y0"=w230:dbl)
              n294 = feedback-in #43(w228) -> ()
              n295 = feedback-in #44(w230) -> ()
              n296 = Subtract(x=w91, y=w230) -> (x-y=w229:dbl)
              n297 = feedback-in #26(w229) -> ()
              n298 = formula code="y0=(2*Tau*(u0-u1)-(T-2*Tau)*y1)/(T+2*Tau);"("Tau"=w322, "u0"=w229, "u1"=w328, "y1"=w330, "T"=0.001 ("input variable")) -> ("y0"=w332:dbl)
              n299 = feedback-in #37(w332) -> ()
              n300 = Multiply(x=w332, y="MFC_FB_gain") -> (x*y=w323:dbl)
              n301 = Select(t=w323, s="MFC", f=0.0) -> (s? t:f=w321:dbl)
              n302 = feedback-in #21(w321) -> ()
              n303 = Subtract(x=w111, y=w228) -> (x-y=w227:dbl)
              n304 = feedback-in #27(w227) -> ()
              n305 = formula code="y0=(2*Tau*(u0-u1)-(T-2*Tau)*y1)/(T+2*Tau);"("Tau"=w322, "u0"=w227, "u1"=w353, "y1"=w351, "T"=0.001 ("input variable")) -> ("y0"=w347:dbl)
              n306 = feedback-in #38(w347) -> ()
              n307 = Multiply(x=w347, y="MFC_FB_gain") -> (x*y=w346:dbl)
              n308 = Select(t=w346, s="MFC", f=0.0) -> (s? t:f=w319:dbl)
              n309 = feedback-in #18(w319) -> ()
              n310 = node-c288() -> ()  [unwired: 1 in, 1 out]
              "now interation" <- w284
            }
            n311 = node-c288(w89) -> ()  [unwired: 1 out]
          }
          frame True {
          }
        }
        n312 = node-c288() -> ()  [unwired: 1 in, 1 out]
      }
      n313 = call <vilib>:"Simple Error Handler.vi"("error in (no error)"=w30) -> ("error out"=w39:errorcluster)  [unwired: 4 in, 4 out]
      n314 = call <vilib>:"Reset myRIO.vi"("error in (no error)"=w39) -> ()  [unwired: 10 in, 1 out]
      n315 = node-c288(w25) -> ()  [unwired: 1 out]
    }
  }
